vi "json parse.vi"() -> ()   [LabVIEW 2014]
panel:
  out "值":string
  out "JSON out":string
  out "匹配之前的子字符串 2":string
  out "匹配+剩余字符串":string
  out "匹配之前的子字符串":string
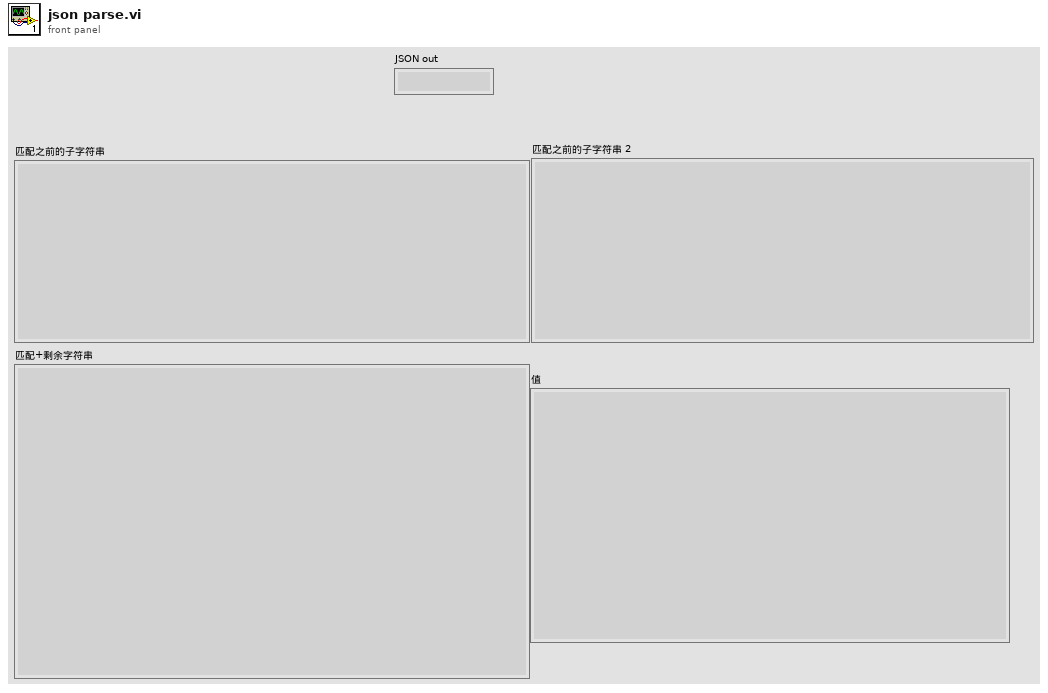
[diagram p1: front panel]
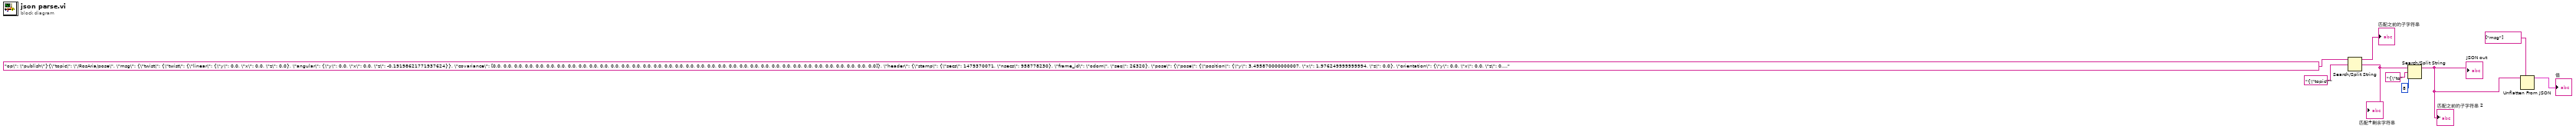
[diagram p0: block diagram]
diagram:
  n1 = Search/Split String(string="op\": \"publish\"}{\"topic\": \"/RosAria/pose\", \"msg\": {\"twist\": {\"twist\": {\"linear\": {\"y\": 0.0, \"x\": 0.0, \"z\": 0.0}, \"angular\": {\"y\": 0.0, \"x\": 0.0, \"z\": -0.19198621771937624}}, \"covariance\": [0.0, 0.0, 0.0, 0.0, 0.0, 0.0, 0.0, 0.0, 0.0, 0.0, 0.0, 0.0, 0.0, 0.0, 0.0, 0.0, 0.0, 0.0, 0.0, 0.0, 0.0, 0.0, 0.0, 0.0, 0.0, 0.0, 0.0, 0.0, 0.0, 0.0, 0.0, 0.0, 0.0, 0.0, 0.0, 0.0]}, \"header\": {\"stamp\": {\"secs\": 1479370071, \"nsecs\": 958778230}, \"frame_id\": \"odom\", \"seq\": 26320}, \"pose\": {\"pose\": {\"position\": {\"y\": 3.495870000000007, \"x\": 1.976249999999994, \"z\": 0.0}, \"orientation\": {\"y\": 0.0, \"x\": 0.0, \"z\": 0.775432651600462, \"w\": 0.6314302834295141}}, \"covariance\": [0.0, 0.0, 0.0, 0.0, 0.0, 0.0, 0.0, 0.0, 0.0, 0.0, 0.0, 0.0, 0.0, 0.0, 0.0, 0.0, 0.0, 0.0, 0.0, 0.0, 0.0, 0.0, 0.0, 0.0, 0.0, 0.0, 0.0, 0.0, 0.0, 0.0, 0.0, 0.0, 0.0, 0.0, 0.0, 0.0]}, \"child_frame_id\": \"base_link\"}, \"op\": \"publish\"}{\"topic\": \"/RosAria/pose\", \"msg\": {\"twist\": {\"twist\": {\"linear\": {\"y\": 0.0, \"x\": 0.0, \"z\": 0.0}, \"angular\": {\"y", search string/char (-)="{\"topic\"" ("搜索字符串")) -> (substring before match=→"匹配之前的子字符串":string, match + rest of string=w6:string)  [unwired: 1 in, 1 out]
  "匹配+剩余字符串" <- w6
  n2 = Search/Split String(string=w6, search string/char (-)="{\"to" ("搜索字符串/字符(-)"), offset (0)=8 ("偏移量(0)")) -> (substring before match=w3:string)  [unwired: 2 out]
  "匹配之前的子字符串 2" <- w3
  "JSON out" <- w3
  n3 = Unflatten From JSON(path=string[] ["msg"] ("路径"), JSON string=w3) -> (value=→"值":cluster{})  [unwired: 5 in, 1 out]
